vi "OpenAC230V_L.vi"(0 "datain":string[](array[string])=["备注", "负载通道", "负载地址", "延时时间", "output max", "output min", "量测类型", "待测物板号"], 5 "HW CH Number":i32, 7 "Setup":string) -> (4 "REPORT INDECATE":string[][](array[string])=[["微安测试", "", "", "", ""], ["微安量测", "4", "0.000", "0.1", "NG"], ["微安量测", "4", "0.000", "0.1", "NG"], ["微安量测", "4", "0.000", "0.1", "NG"], ["微安量测", "4", "0.000", "0.1", "NG"]], 6 "ROW HEAD":string[](array[string]), 8 "PF":string[](array[string]), 10 "testData":string[](array[string]), 15 "Array":string[](array[string]))   [LabVIEW 2018]
uses:
  Subvi/Global.vi
panel:
  out "测试板数":i32
  out "数组":bool[](array[boolean])
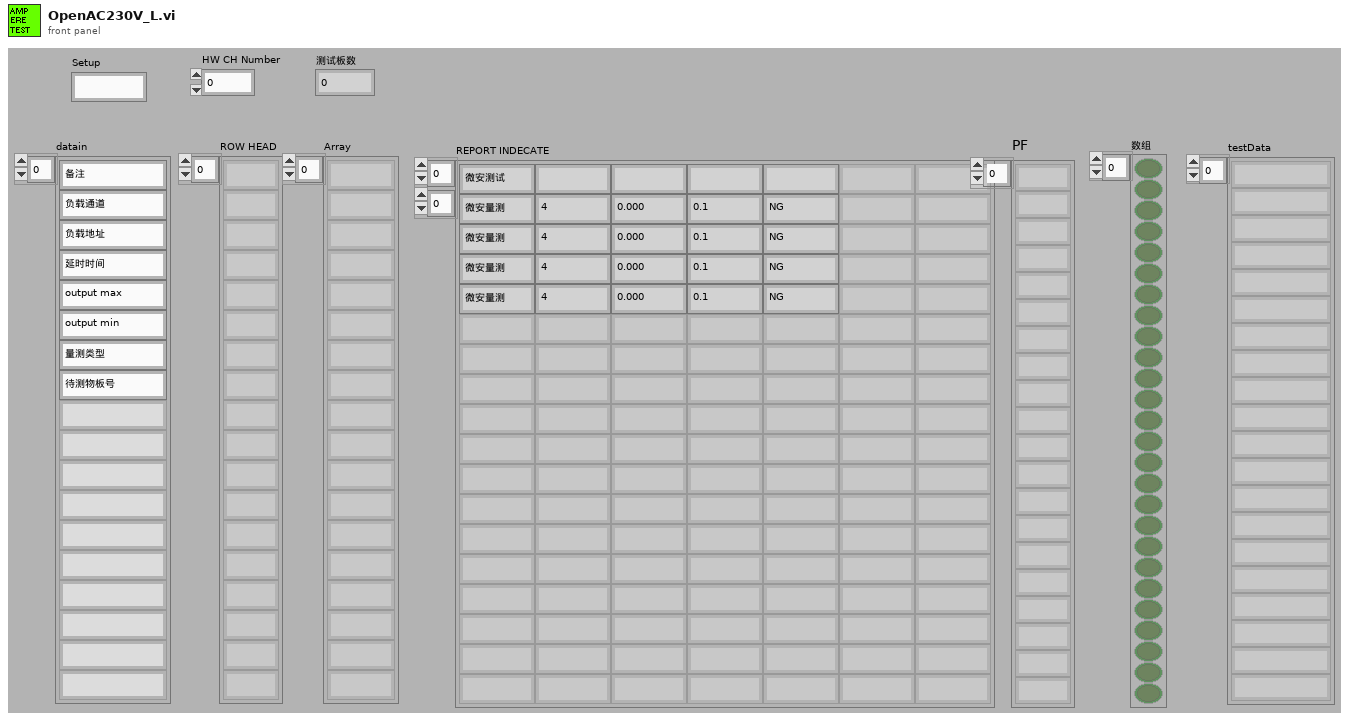
[diagram p1: front panel]
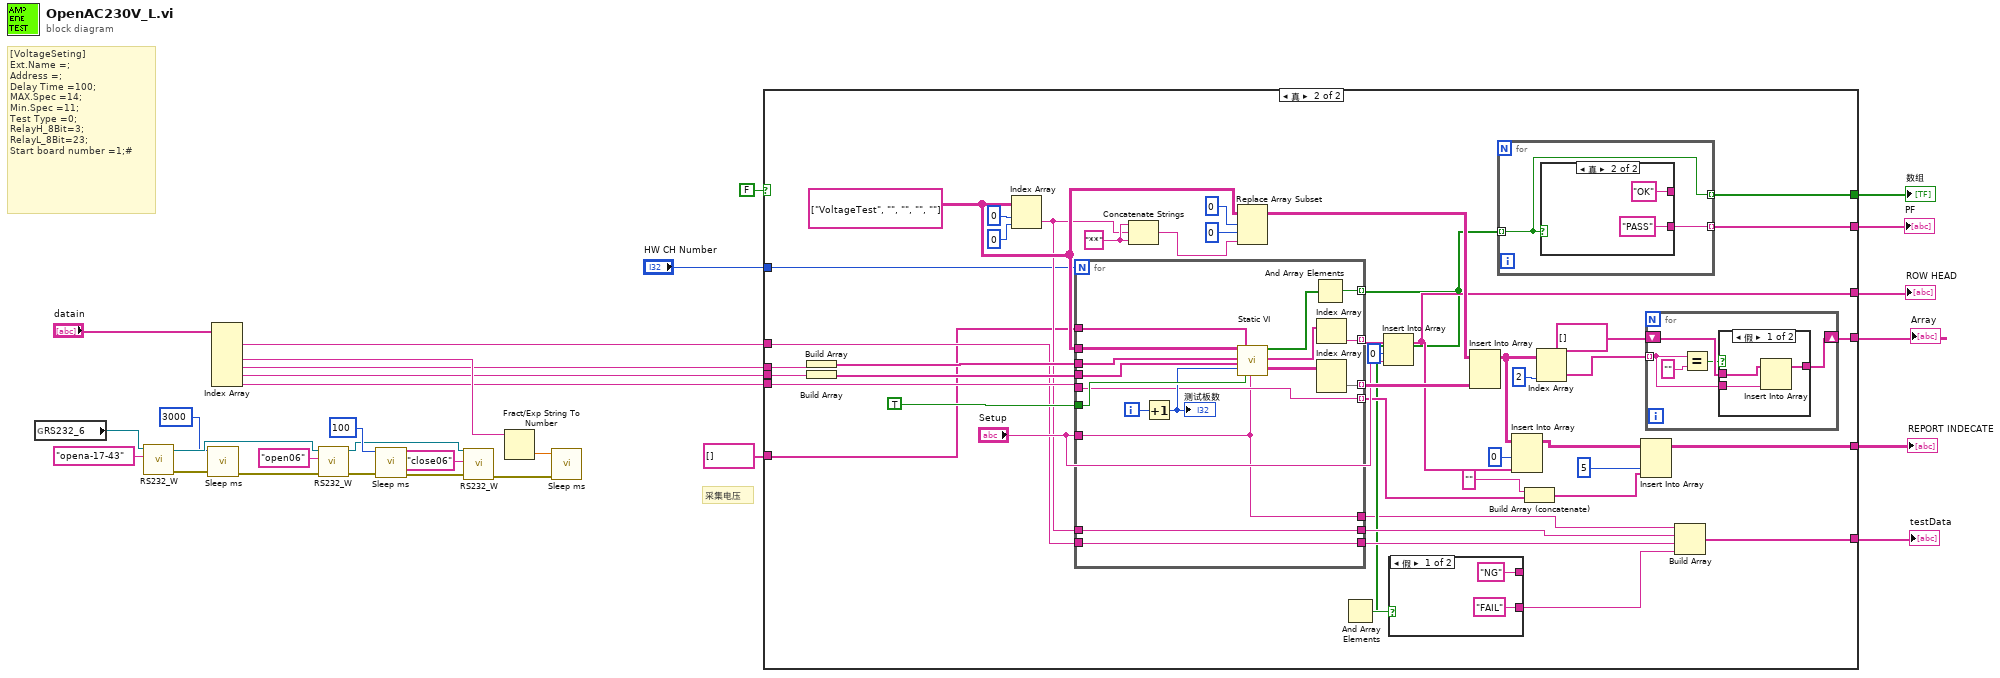
[diagram p0: block diagram]
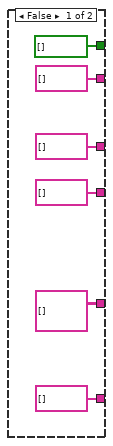
[diagram p2: hidden frame]
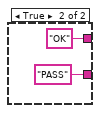
[diagram p3: hidden frame]
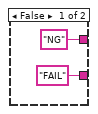
[diagram p4: hidden frame]
diagram:
  # "采集电压"
  # "[VoltageSeting]\nExt.Name =;\nAddress =;\nDelay Time =100;\nMAX.Spec =14;\nMin.Spec =11;\nTest Type =0;\nRelayH_8Bit=3;\nRelayL_8Bit=23;\nStart board number =1;#"
  n1 = global read "Global.vi" "RS232_6"() -> (w15:refnum<visa-resource-name>)
  n2 = call "RS232_W.vi"("CMD"="opena-17-43", "VISA资源名称"=w15) -> ("error out"=w3:errorcluster, "VISA资源名称输出"=w4:refnum<visa-resource-name>)  [unwired: 7 in, 1 out]
  n3 = call "Sleep ms.vi"("error in (no error)"=w3, "等待时间（毫秒）"=u32 3000) -> ("error out"=w5:errorcluster)  [unwired: 9 in]
  n4 = Index Array(array="datain") -> (element #1=w20:string, element #3=w26:string, element #4=w25:string, element #5=w24:string, element #6=w22:string)  [unwired: 6 in, 1 out]
  n5 = call "RS232_W.vi"("error in (no error)"=w5, "CMD"="open06", "VISA资源名称"=w4) -> ("error out"=w11:errorcluster, "VISA资源名称输出"=w7:refnum<visa-resource-name>)  [unwired: 6 in, 1 out]
  n6 = call "Sleep ms.vi"("error in (no error)"=w11, "等待时间（毫秒）"=u32 100) -> ("error out"=w8:errorcluster)  [unwired: 9 in]
  n7 = call "RS232_W.vi"("error in (no error)"=w8, "CMD"="close06", "VISA资源名称"=w7) -> ("error out"=w6:errorcluster)  [unwired: 6 in, 2 out]
  n8 = Fract/Exp String To Number(string=w26) -> (number=w16:dbl)  [unwired: 3 in, 1 out]
  n9 = call "Sleep ms.vi"("error in (no error)"=w6, "等待时间（毫秒）"=w16) -> ()  [unwired: 9 in, 1 out]
  n10 = case shown="真" FALSE {
    tunnel: [string[] [] ("Array") w76] -> w29
    tunnel: [string[] [] w75] -> w28
    tunnel: w25 -> [_ w68]
    tunnel: w24 -> [_ w67]
    tunnel: [string[] [] w56] -> w23
    tunnel: w22 -> [_ w54]
    tunnel: [string[][] [] w51] -> w21
    tunnel: w20 -> [_ w46]
    tunnel: [string[] [] w40] -> w19
    tunnel: [bool[] [] w38] -> w18
    tunnel: "HW CH Number" -> [_ w37]
    tunnel: string[] [] ("Out data") -> [_ w36]
    frame False {
    }
    frame True {
      w66 = string[][] [["VoltageTest", "", "", "", ""]]
      w72 = "**" ("字符串")
      n11 = Build Array(w68) -> (w65:string[])
      n12 = Build Array(w67) -> (w64:string[])
      n13 = Index Array(array=w66, index (row)=0 ("索引 (行)"), index (col)=0 ("禁用的索引 (列)")) -> (element=w47:string)
      n14 = for {
        N: w37 -> [_]
        tunnel: w36 -> [w100]
        tunnel: w65 -> [w98]
        tunnel: w64 -> [w97]
        tunnel: "Setup" -> [w84]
        tunnel: TRUE -> [w95]
        tunnel: [w93] -> w42 mode=indexing
        tunnel: [w90] -> w60 mode=indexing
        tunnel: w66 -> [w99]
        tunnel: [w88] -> w61 mode=indexing
        tunnel: w54 -> [w87]
        tunnel: [w87] -> w50 mode=indexing
        tunnel: w47 -> [w86]
        tunnel: [w86] -> w45
        tunnel: w46 -> [w85]
        tunnel: [w85] -> w44
        tunnel: [w84] -> w39
        i -> [w92]
        n15 = Increment(x=w92) -> (x+1=w94:i32)
        "测试板数" <- w94
        n16 = call "Static VI.vi"("添加的数组"=w99, "Max"=w98, "Min"=w97, "板数"=w94, "INPUTSTRING"=w100, "是否为字符串对比"=w95, "SQ"=w84) -> ("P/F"=w96:bool[], "SQ out"=w91:string[], "arrauy out"=w89:string[][])  [unwired: 9 in, 1 out]
        n17 = And Array Elements(Boolean array=w96) -> (logical AND=w93:bool)
        n18 = Index Array(array=w91) -> (element=w90:string)  [unwired: 1 in]
        n19 = Index Array(array=w89) -> (element=w88:string[])  [unwired: 2 in]
      }
      n20 = Concatenate Strings(w72, w47, w72) -> (w69:string)
      n21 = Replace Array Subset(array=w66, new element=w69, index (row)=0 ("索引 (行)"), index (col)=0 ("禁用的索引 (列)")) -> (w62:string[][])
      n22 = And Array Elements(Boolean array=w42) -> (logical AND=w43:bool)
      n23 = Insert Into Array(array=w60, index=0 ("索引"), new element="Setup") -> (w56:string[])
      n24 = case shown="假" w43 {
        tunnel: ["NG" "OK"] -> _
        tunnel: ["FAIL" "PASS"] -> w41
        frame False {
        }
        frame True {
        }
      }
      n25 = Insert Into Array ("数组插入")(array=w62, new element=w61) -> (w57:string[][])  [unwired: 2 in]
      n26 = for {
        tunnel: w42 -> [w101] mode=indexing
        tunnel: [w102] -> w75 mode=indexing
        tunnel: [w101] -> w38 mode=indexing
        n27 = case shown="真" w101 {
          tunnel: ["NG" "OK"] -> _
          tunnel: ["FAIL" "PASS"] -> w102
          frame False {
          }
          frame True {
          }
        }
      }
      n28 = Insert Into Array(array=w57, index (col)=0 ("禁用的索引 (列)"), new element=w56) -> (w52:string[][])  [unwired: 1 in]
      n29 = Build Array (concatenate)("" ("字符串"), w50) -> (w48:string[])
      n30 = Index Array(array=w57, index (col)=2 ("禁用的索引 (列)")) -> (element=w77:string[])  [unwired: 1 in]
      n31 = Insert Into Array(array=w52, index (col)=5 ("禁用的索引 (列)"), new element=w48) -> (w51:string[][])  [unwired: 1 in]
      n32 = for {
        tunnel: w77 -> [w107] mode=indexing
        shift-right: [w108] -> w76
        shift-left: string[] [] ("Array") -> [w111]
        n33 = Equal?(x=w107, y="") -> (x = y?=w109:bool)
        n34 = case shown="假" w109 {
          tunnel: w111 -> [w114 w115]
          tunnel: [w113 w115] -> w108
          tunnel: w107 -> [w112 _]
          frame False {
            n35 = Insert Into Array(array=w114, new element=w112) -> (w113:string[])  [unwired: 1 in]
          }
          frame True {
          }
        }
      }
      n36 = Build Array(w39, w45, w44, w41) -> (w40:string[])
    }
  }
  "REPORT INDECATE" <- w21
  "ROW HEAD" <- w23
  "PF" <- w28
  "Array" <- w29
  "数组" <- w18
  "testData" <- w19
